vi "Set Default if Unwired.vi"(8 "error in (no error)":errorcluster, 11 "VI Path":path) -> (0 "error out":errorcluster)   [LabVIEW 2016, in "SLL Scripting.lvlib" / "SLL Class DVR API Generator.lvlib"]
uses:
  SLL Class DVR API Generator.lvlib
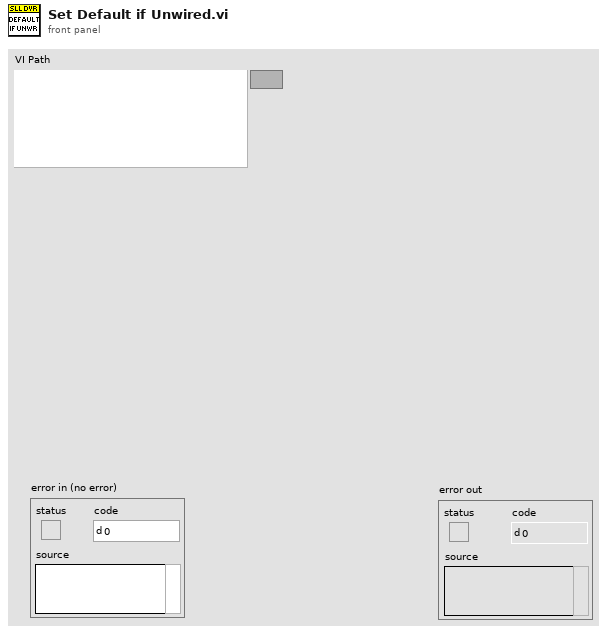
[diagram p1: front panel]
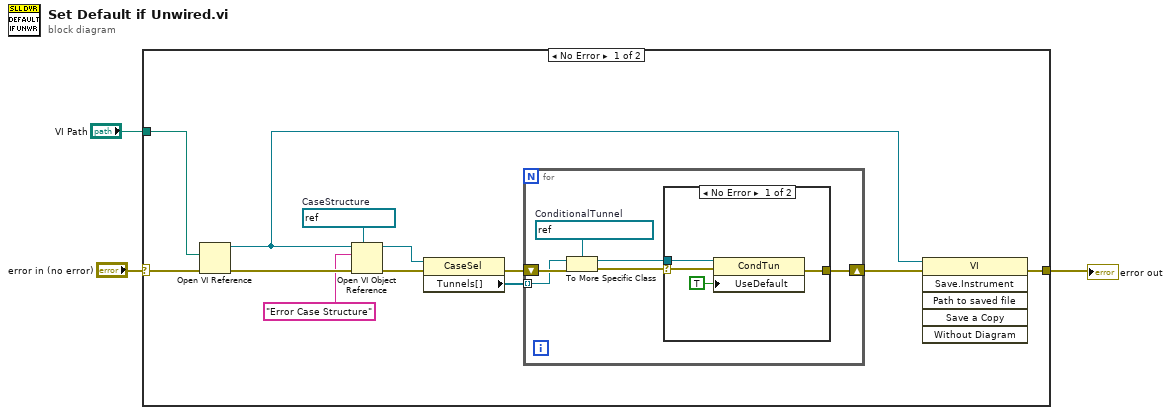
[diagram p0: block diagram]
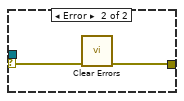
[diagram p2: hidden frame]
diagram:
  n1 = case shown="No Error" "error in (no error)" {
    selector: "error in (no error)" -> [w15 w28]
    tunnel: [w5 w28] -> w2
    tunnel: "VI Path" -> [w7 _]
    frame No Error {
      w11 = refnum<vi> refnum  # CaseStructure
      n2 = Open VI Reference(vi path=w7, error in (no error)=w15) -> (vi reference=w4:refnum<vi>, error out=w14:errorcluster)  [unwired: 4 in]
      n3 = Open VI Object Reference(7:w11, 8:w14, 10:"Error Case Structure" ("name/order"), 11:w4) -> (0:w13:errorcluster, 3:w6:refnum<vi>)
      n4 = property class="CaseSel"(reference=w6, error in=w13) -> (error out=w10:errorcluster, "Tunnels[]"=w8:refnum<vi>[])  [unwired: 1 out]
      n5 = for {
        shift-right: [w17] -> w9
        shift-left: w10 -> [w21]
        tunnel: w8 -> [w20] mode=indexing
        w19 = refnum<vi> refnum  # ConditionalTunnel
        n6 = To More Specific Class(target class=w19, reference=w20, error in=w21) -> (specific class reference=w18:refnum<vi>, error out=w16:errorcluster)
        n7 = case shown="No Error" w16 {
          selector: w16 -> [w23 w27]
          tunnel: w18 -> [w25 _]
          tunnel: [w24 w26] -> w17
          frame No Error {
            n8 = property class="CondTun"(reference=w25, error in=w23, "UseDefault"=TRUE ("Use Default if Unwired")) -> (error out=w24:errorcluster)  [unwired: 1 out]
          }
          frame Error {
            n9 = call <vilib>:"Clear Errors.vi"("error in (no error)"=w27) -> ("error out"=w26:errorcluster)  [unwired: 5 in, 1 out]
          }
        }
      }
      n10 = invoke class="VI" method="Save.Instrument"(reference=w4, error in=w9) -> (error out=w5:errorcluster)  [unwired: 4 in, 5 out]
    }
    frame Error {
    }
  }
  "error out" <- w2
